vi "Sort References By Type.vi"(10 "Controls to Register":refnum<vi>[](array[refnum])) -> (2 "Controls":T1)   [LabVIEW 2015, in "AutoRegistration.lvlib" / "AutoRegistration.lvclass"]
uses:
  AutoRegistration.lvclass
  Registration References.ctl
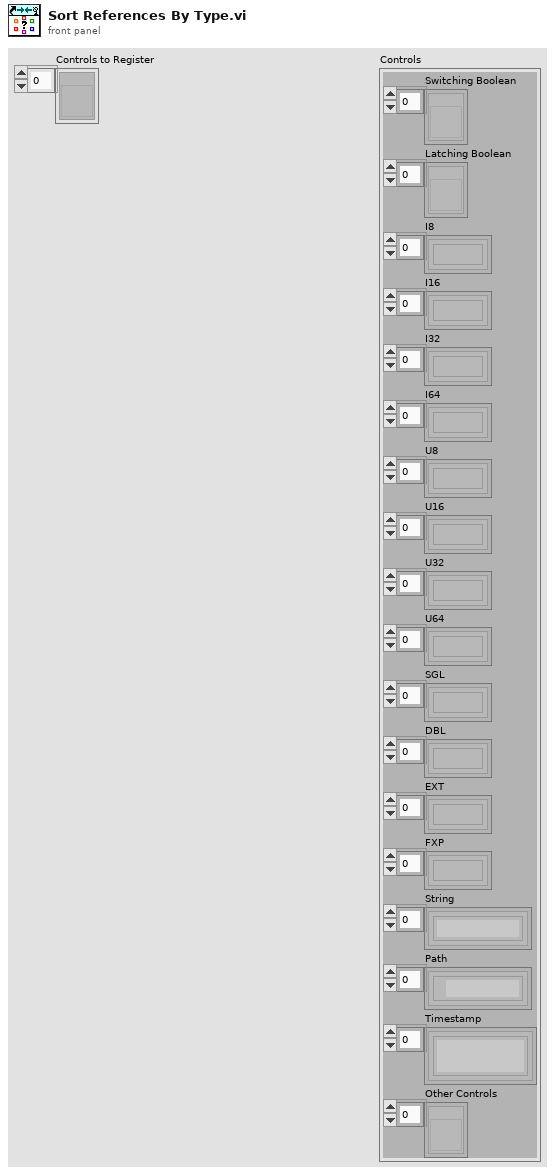
[diagram p1: front panel]
types:
  T1 = typedef "AutoRegistration.lvlib/AutoRegistration.lvclass/Registration References.ctl" = cluster{"Switching Boolean":refnum<vi>[], "Latching Boolean":refnum<vi>[], "I8":refnum<vi>[], "I16":refnum<vi>[], "I32":refnum<vi>[], "I64":refnum<vi>[], "U8":refnum<vi>[], "U16":refnum<vi>[], "U32":refnum<vi>[], "U64":refnum<vi>[], "SGL":refnum<vi>[], "DBL":refnum<vi>[], "EXT":refnum<vi>[], "FXP":refnum<vi>[], "String":refnum<vi>[], "Path":refnum<vi>[], "Timestamp":refnum<vi>[], "Other Controls":refnum<vi>[]}
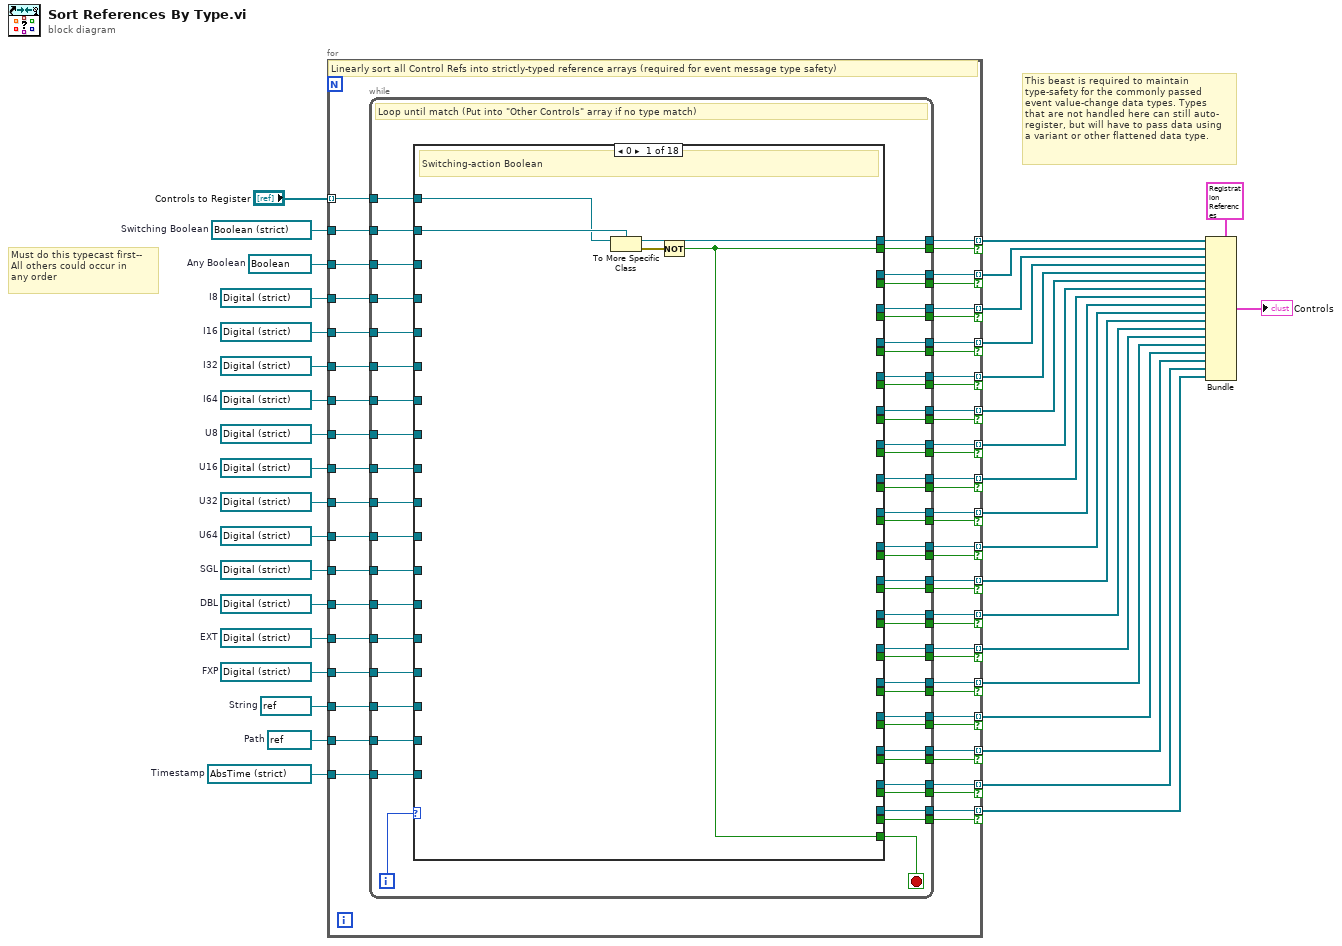
[diagram p0: block diagram]
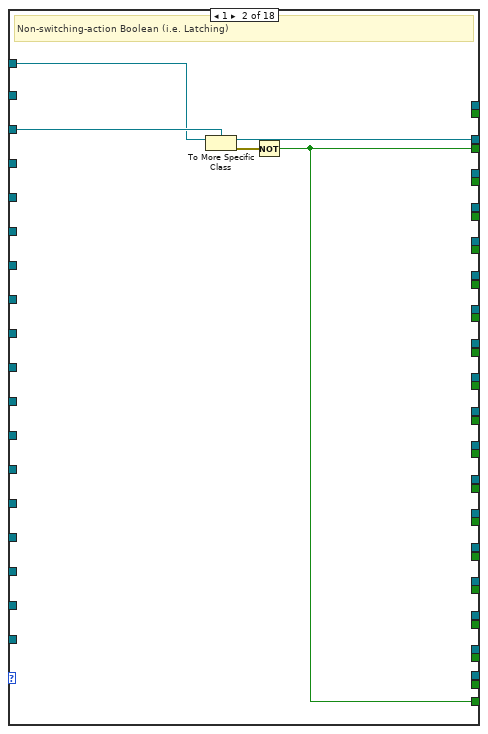
[diagram p2: hidden frame]
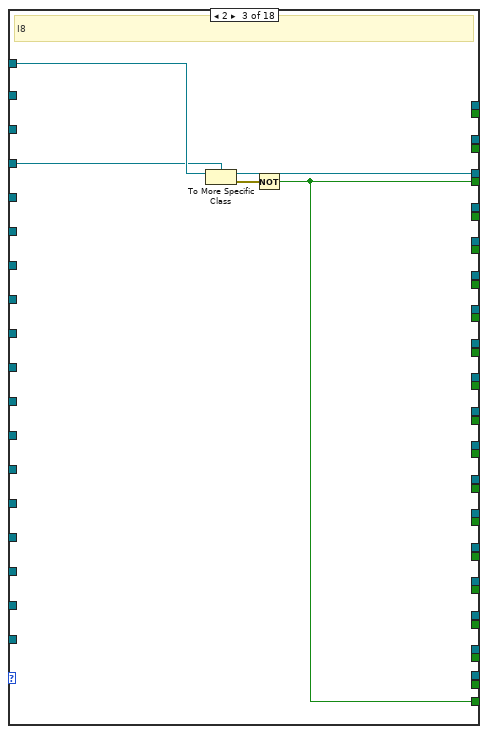
[diagram p3: hidden frame]
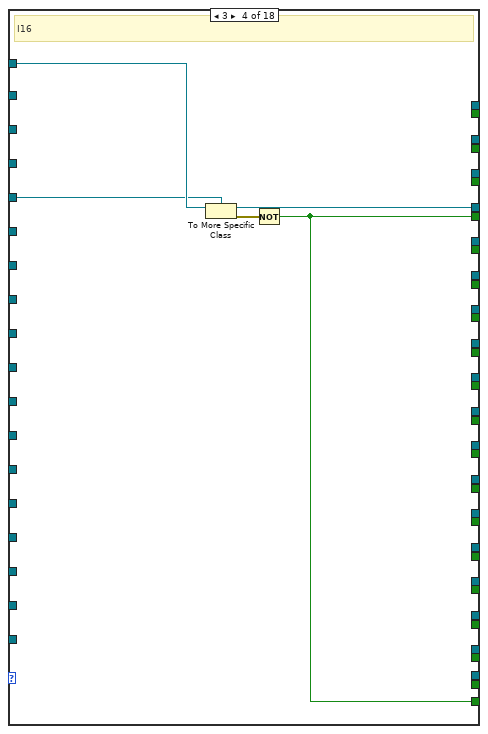
[diagram p4: hidden frame]
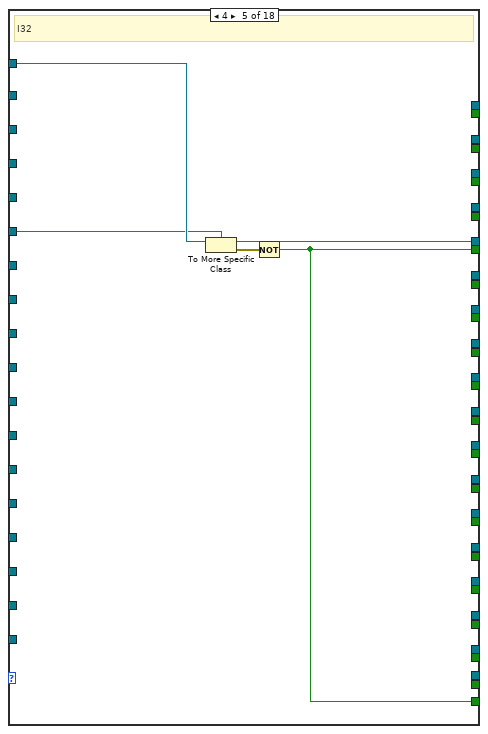
[diagram p5: hidden frame]
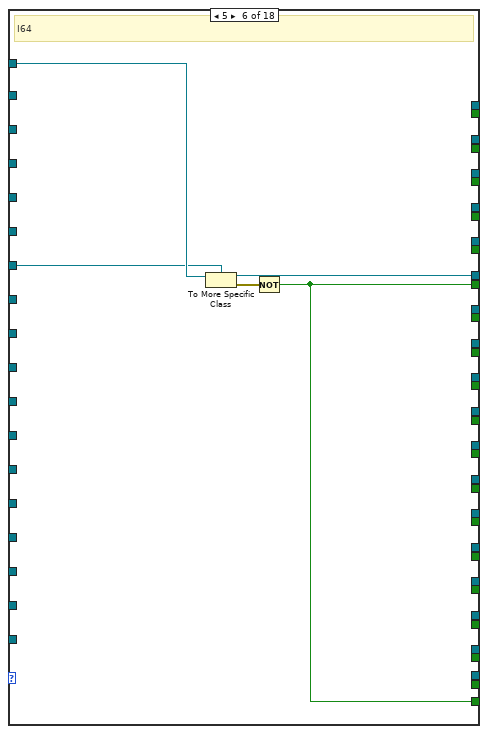
[diagram p6: hidden frame]
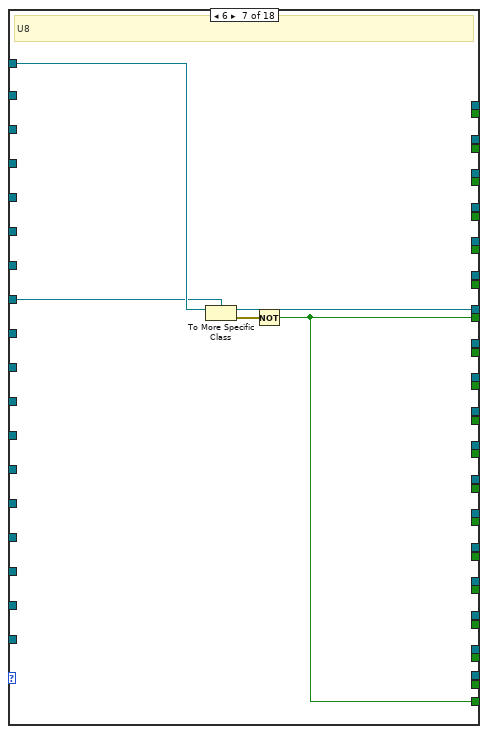
[diagram p7: hidden frame]
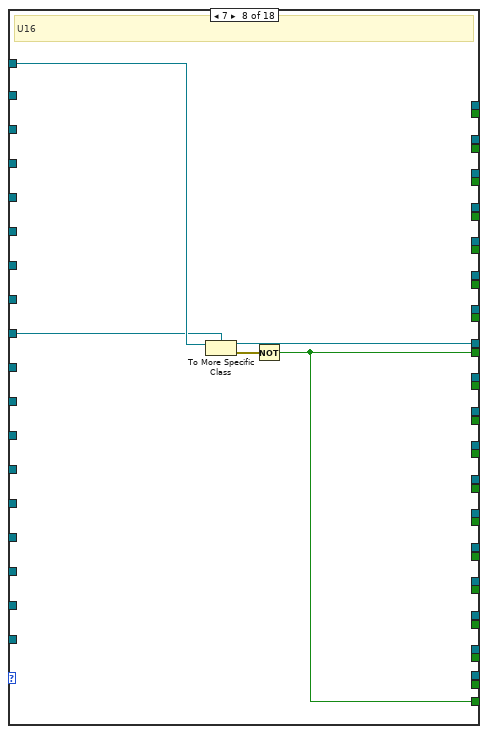
[diagram p8: hidden frame]
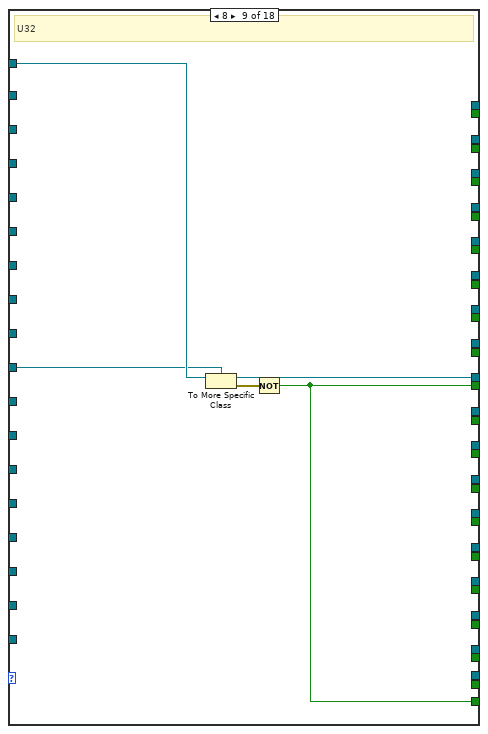
[diagram p9: hidden frame]
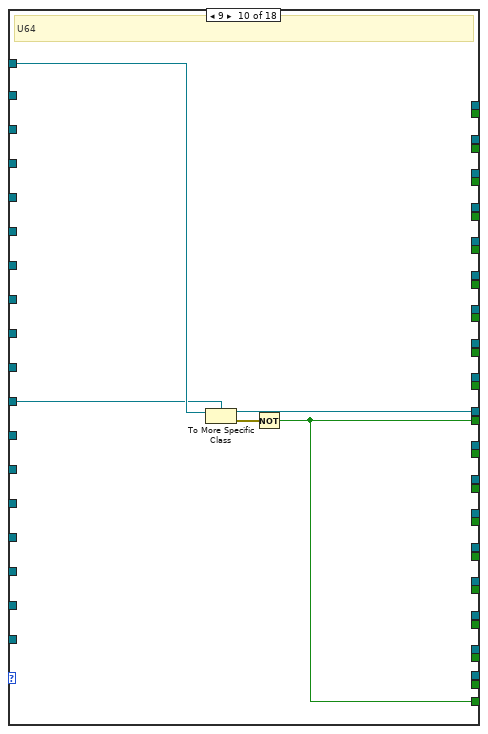
[diagram p10: hidden frame]
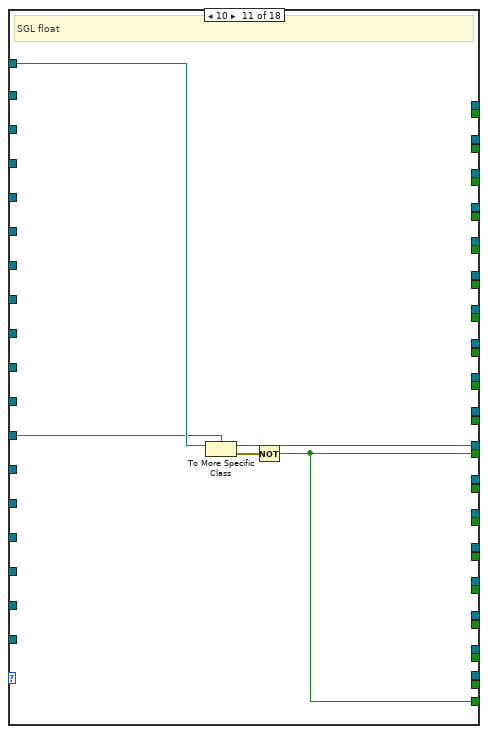
[diagram p11: hidden frame]
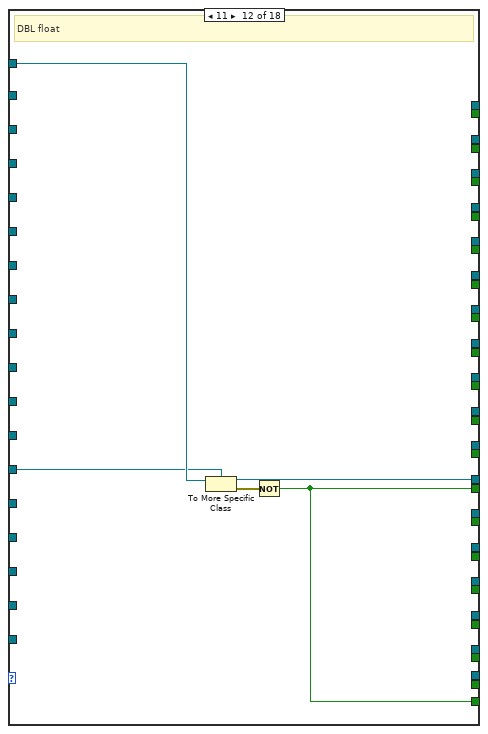
[diagram p12: hidden frame]
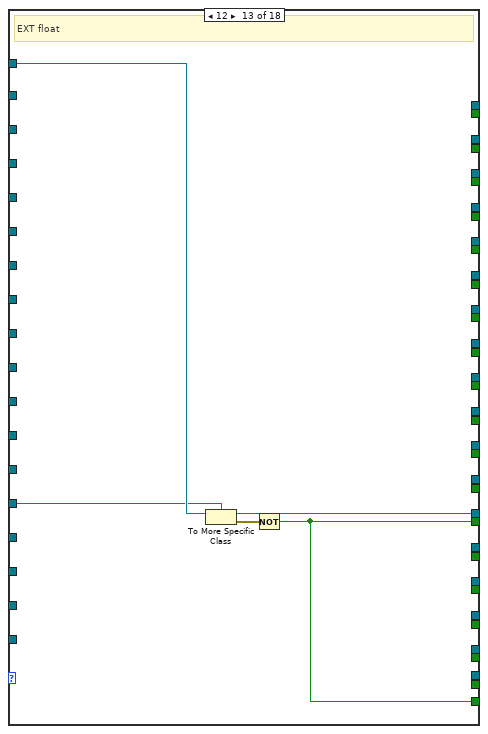
[diagram p13: hidden frame]
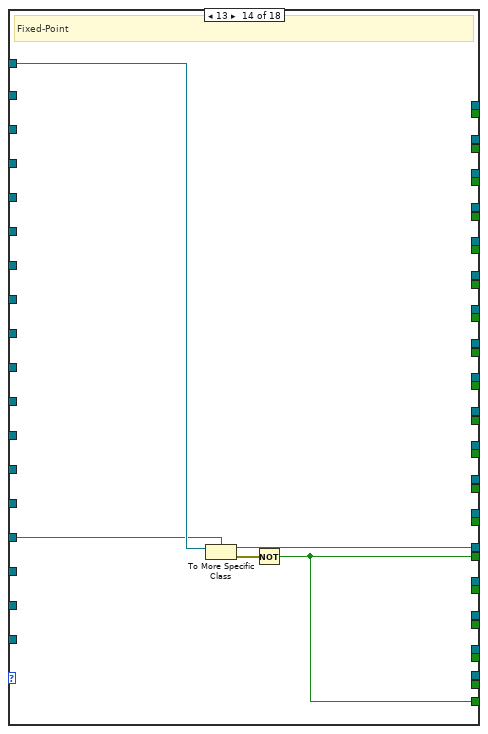
[diagram p14: hidden frame]
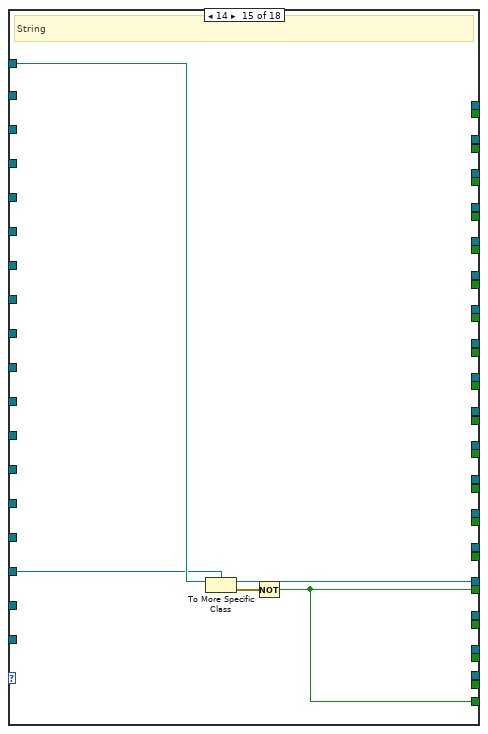
[diagram p15: hidden frame]
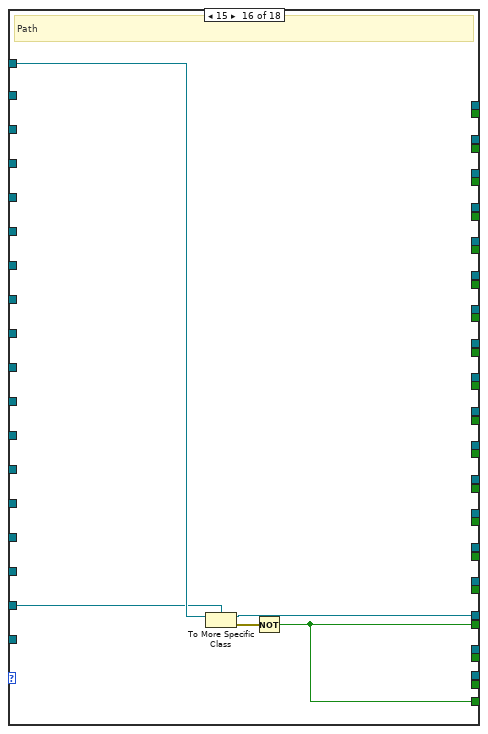
[diagram p16: hidden frame]
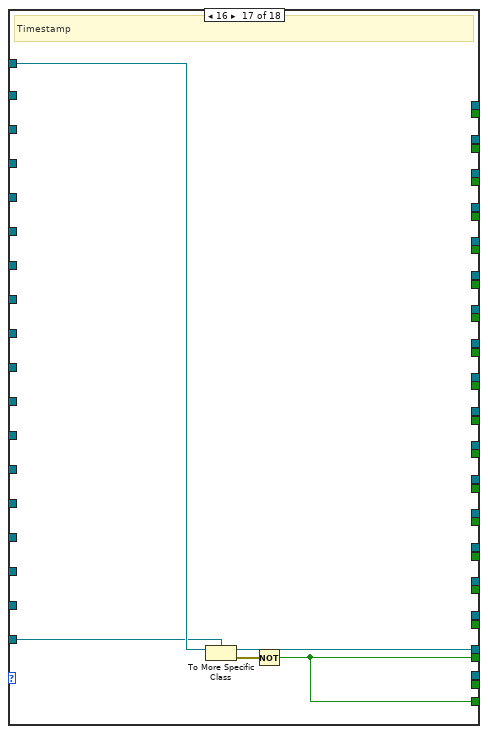
[diagram p17: hidden frame]
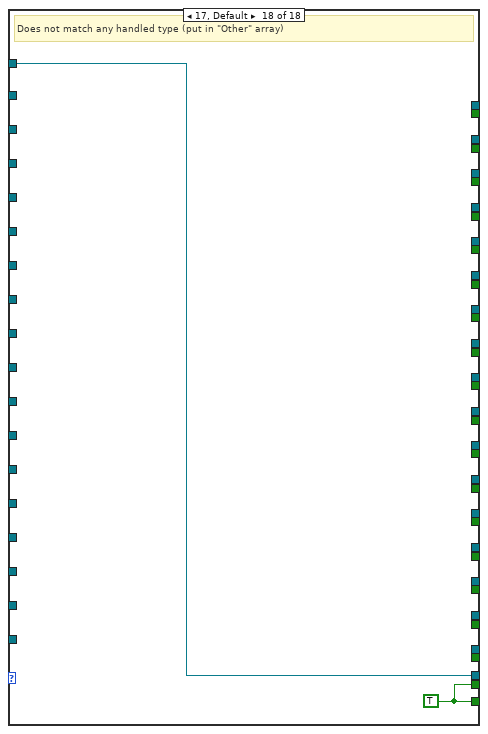
[diagram p18: hidden frame]
diagram:
  w21 = refnum<vi> refnum  # Switching Boolean
  w22 = refnum<vi> refnum  # Any Boolean
  w23 = refnum<vi> refnum  # I8
  w24 = refnum<vi> refnum  # I16
  w25 = refnum<vi> refnum  # I32
  w26 = refnum<vi> refnum  # I64
  w27 = refnum<vi> refnum  # U8
  w28 = refnum<vi> refnum  # U16
  w29 = refnum<vi> refnum  # U32
  w30 = refnum<vi> refnum  # U64
  w31 = refnum<vi> refnum  # SGL
  w32 = refnum<vi> refnum  # DBL
  w33 = refnum<vi> refnum  # EXT
  w34 = refnum<vi> refnum  # FXP
  w35 = refnum<vi> refnum  # String
  w36 = refnum<vi> refnum  # Path
  w37 = refnum<vi> refnum  # Timestamp
  # "Must do this typecast first--\nAll others could occur in\nany order"
  # "This beast is required to maintain\ntype-safety for the commonly passed\nevent value-change data types. Types\nthat are not handled here can still auto-\nregister, but will have to pass data using\na variant or other flattened data type."
  n1 = for {
    tunnel: "Controls to Register" -> [w41] mode=indexing
    tunnel: w37 -> [w92]
    tunnel: w36 -> [w91]
    tunnel: w35 -> [w90]
    tunnel: w34 -> [w89]
    tunnel: w33 -> [w88]
    tunnel: w32 -> [w87]
    tunnel: w31 -> [w86]
    tunnel: w30 -> [w85]
    tunnel: w29 -> [w84]
    tunnel: w28 -> [w83]
    tunnel: w27 -> [w82]
    tunnel: w26 -> [w81]
    tunnel: w25 -> [w80]
    tunnel: w24 -> [w79]
    tunnel: w23 -> [w78]
    tunnel: w22 -> [w77]
    tunnel: w21 -> [w76]
    tunnel: [w75] -> w20 mode=indexing if=w42
    tunnel: [w74] -> w19 mode=indexing if=w58
    tunnel: [w73] -> w18 mode=indexing if=w43
    tunnel: [w72] -> w17 mode=indexing if=w44
    tunnel: [w71] -> w16 mode=indexing if=w45
    tunnel: [w70] -> w15 mode=indexing if=w46
    tunnel: [w69] -> w14 mode=indexing if=w47
    tunnel: [w68] -> w13 mode=indexing if=w48
    tunnel: [w67] -> w12 mode=indexing if=w49
    tunnel: [w66] -> w11 mode=indexing if=w50
    tunnel: [w65] -> w10 mode=indexing if=w51
    tunnel: [w64] -> w9 mode=indexing if=w52
    tunnel: [w63] -> w8 mode=indexing if=w53
    tunnel: [w62] -> w7 mode=indexing if=w54
    tunnel: [w61] -> w6 mode=indexing if=w55
    tunnel: [w60] -> w5 mode=indexing if=w56
    tunnel: [w59] -> w4 mode=indexing if=w57
    tunnel: [w40] -> w3 mode=indexing if=w39
    # "Linearly sort all Control Refs into strictly-typed reference arrays (required for event message type safety)"
    n2 = while {
      tunnel: [w114] -> w58
      tunnel: [w113] -> w57
      tunnel: [w112] -> w56
      tunnel: [w111] -> w55
      tunnel: [w110] -> w54
      tunnel: [w109] -> w53
      tunnel: [w108] -> w52
      tunnel: [w107] -> w51
      tunnel: [w106] -> w50
      tunnel: [w105] -> w49
      tunnel: [w104] -> w48
      tunnel: [w103] -> w47
      tunnel: [w102] -> w46
      tunnel: [w101] -> w45
      tunnel: [w100] -> w44
      tunnel: [w99] -> w43
      tunnel: [w98] -> w42
      tunnel: w41 -> [w97]
      tunnel: w76 -> [w132]
      tunnel: [w131] -> w75
      tunnel: w77 -> [w133]
      tunnel: [w130] -> w74
      tunnel: w78 -> [w134]
      tunnel: [w129] -> w73
      tunnel: w79 -> [w135]
      tunnel: [w128] -> w72
      tunnel: w80 -> [w136]
      tunnel: [w127] -> w71
      tunnel: w81 -> [w137]
      tunnel: [w126] -> w70
      tunnel: w82 -> [w138]
      tunnel: [w125] -> w69
      tunnel: w83 -> [w139]
      tunnel: [w124] -> w68
      tunnel: w84 -> [w140]
      tunnel: [w123] -> w67
      tunnel: w85 -> [w141]
      tunnel: [w122] -> w66
      tunnel: w86 -> [w142]
      tunnel: [w121] -> w65
      tunnel: w87 -> [w143]
      tunnel: [w120] -> w64
      tunnel: w88 -> [w144]
      tunnel: [w119] -> w63
      tunnel: w89 -> [w145]
      tunnel: [w118] -> w62
      tunnel: w90 -> [w146]
      tunnel: [w117] -> w61
      tunnel: w91 -> [w147]
      tunnel: [w116] -> w60
      tunnel: w92 -> [w148]
      tunnel: [w115] -> w59
      tunnel: [w94] -> w40
      tunnel: [w93] -> w39
      i -> [w95]
      stop <- w96 stop-if-true
      # "Loop until match (Put into \"Other Controls\" array if no type match)"
      n3 = case shown="0" w95 {
        tunnel: w148 -> [_ _ _ _ _ _ _ _ _ _ _ _ _ _ _ _ w229 _]
        tunnel: w147 -> [_ _ _ _ _ _ _ _ _ _ _ _ _ _ _ w224 _ _]
        tunnel: w146 -> [_ _ _ _ _ _ _ _ _ _ _ _ _ _ w219 _ _ _]
        tunnel: w145 -> [_ _ _ _ _ _ _ _ _ _ _ _ _ w216 _ _ _ _]
        tunnel: w144 -> [_ _ _ _ _ _ _ _ _ _ _ _ w211 _ _ _ _ _]
        tunnel: w143 -> [_ _ _ _ _ _ _ _ _ _ _ w206 _ _ _ _ _ _]
        tunnel: w142 -> [_ _ _ _ _ _ _ _ _ _ w201 _ _ _ _ _ _ _]
        tunnel: w141 -> [_ _ _ _ _ _ _ _ _ w196 _ _ _ _ _ _ _ _]
        tunnel: w140 -> [_ _ _ _ _ _ _ _ w191 _ _ _ _ _ _ _ _ _]
        tunnel: w139 -> [_ _ _ _ _ _ _ w186 _ _ _ _ _ _ _ _ _ _]
        tunnel: w138 -> [_ _ _ _ _ _ w181 _ _ _ _ _ _ _ _ _ _ _]
        tunnel: w137 -> [_ _ _ _ _ w174 _ _ _ _ _ _ _ _ _ _ _ _]
        tunnel: w136 -> [_ _ _ _ w171 _ _ _ _ _ _ _ _ _ _ _ _ _]
        tunnel: w135 -> [_ _ _ w166 _ _ _ _ _ _ _ _ _ _ _ _ _ _]
        tunnel: w134 -> [_ _ w160 _ _ _ _ _ _ _ _ _ _ _ _ _ _ _]
        tunnel: w133 -> [_ w158 _ _ _ _ _ _ _ _ _ _ _ _ _ _ _ _]
        tunnel: w132 -> [w153 _ _ _ _ _ _ _ _ _ _ _ _ _ _ _ _ _]
        tunnel: [w152 _ _ _ _ _ _ _ _ _ _ _ _ _ _ _ _ _] -> w131
        tunnel: [_ w154 _ _ _ _ _ _ _ _ _ _ _ _ _ _ _ _] -> w130
        tunnel: [_ _ w159 _ _ _ _ _ _ _ _ _ _ _ _ _ _ _] -> w129
        tunnel: [_ _ _ w165 _ _ _ _ _ _ _ _ _ _ _ _ _ _] -> w128
        tunnel: [_ _ _ _ w169 _ _ _ _ _ _ _ _ _ _ _ _ _] -> w127
        tunnel: [_ _ _ _ _ w175 _ _ _ _ _ _ _ _ _ _ _ _] -> w126
        tunnel: [_ _ _ _ _ _ w179 _ _ _ _ _ _ _ _ _ _ _] -> w125
        tunnel: [_ _ _ _ _ _ _ w184 _ _ _ _ _ _ _ _ _ _] -> w124
        tunnel: [_ _ _ _ _ _ _ _ w189 _ _ _ _ _ _ _ _ _] -> w123
        tunnel: [_ _ _ _ _ _ _ _ _ w194 _ _ _ _ _ _ _ _] -> w122
        tunnel: [_ _ _ _ _ _ _ _ _ _ w199 _ _ _ _ _ _ _] -> w121
        tunnel: [_ _ _ _ _ _ _ _ _ _ _ w204 _ _ _ _ _ _] -> w120
        tunnel: [_ _ _ _ _ _ _ _ _ _ _ _ w209 _ _ _ _ _] -> w119
        tunnel: [_ _ _ _ _ _ _ _ _ _ _ _ _ w214 _ _ _ _] -> w118
        tunnel: [_ _ _ _ _ _ _ _ _ _ _ _ _ _ w220 _ _ _] -> w117
        tunnel: [_ _ _ _ _ _ _ _ _ _ _ _ _ _ _ w225 _ _] -> w116
        tunnel: [_ _ _ _ _ _ _ _ _ _ _ _ _ _ _ _ w230 _] -> w115
        tunnel: [_ w155 _ _ _ _ _ _ _ _ _ _ _ _ _ _ _ _] -> w114
        tunnel: [_ _ _ _ _ _ _ _ _ _ _ _ _ _ _ _ w231 _] -> w113
        tunnel: [_ _ _ _ _ _ _ _ _ _ _ _ _ _ _ w226 _ _] -> w112
        tunnel: [_ _ _ _ _ _ _ _ _ _ _ _ _ _ w221 _ _ _] -> w111
        tunnel: [_ _ _ _ _ _ _ _ _ _ _ _ _ w215 _ _ _ _] -> w110
        tunnel: [_ _ _ _ _ _ _ _ _ _ _ _ w210 _ _ _ _ _] -> w109
        tunnel: [_ _ _ _ _ _ _ _ _ _ _ w205 _ _ _ _ _ _] -> w108
        tunnel: [_ _ _ _ _ _ _ _ _ _ w200 _ _ _ _ _ _ _] -> w107
        tunnel: [_ _ _ _ _ _ _ _ _ w195 _ _ _ _ _ _ _ _] -> w106
        tunnel: [_ _ _ _ _ _ _ _ w190 _ _ _ _ _ _ _ _ _] -> w105
        tunnel: [_ _ _ _ _ _ _ w185 _ _ _ _ _ _ _ _ _ _] -> w104
        tunnel: [_ _ _ _ _ _ w180 _ _ _ _ _ _ _ _ _ _ _] -> w103
        tunnel: [_ _ _ _ _ w176 _ _ _ _ _ _ _ _ _ _ _ _] -> w102
        tunnel: [_ _ _ _ w170 _ _ _ _ _ _ _ _ _ _ _ _ _] -> w101
        tunnel: [_ _ _ w164 _ _ _ _ _ _ _ _ _ _ _ _ _ _] -> w100
        tunnel: [_ _ w161 _ _ _ _ _ _ _ _ _ _ _ _ _ _ _] -> w99
        tunnel: [w149 _ _ _ _ _ _ _ _ _ _ _ _ _ _ _ _ _] -> w98
        tunnel: w97 -> [w150 w156 w162 w167 w172 w177 w182 w187 w192 w197 w202 w207 w212 w217 w222 w227 w232 w235]
        tunnel: [w149 w155 w161 w164 w170 w176 w180 w185 w190 w195 w200 w205 w210 w215 w221 w226 w231 w234] -> w96
        tunnel: [_ _ _ _ _ _ _ _ _ _ _ _ _ _ _ _ _ w235] -> w94
        tunnel: [_ _ _ _ _ _ _ _ _ _ _ _ _ _ _ _ _ w234] -> w93
        frame 0 {
          # "Switching-action Boolean"
          n4 = To More Specific Class(target class=w153, reference=w150) -> (specific class reference=w152:refnum<vi>, error out=w151:errorcluster)  [unwired: 1 in]
          n5 = Not(x=w151) -> (.not. x?=w149:bool)
        }
        frame 1 {
          # "Non-switching-action Boolean (i.e. Latching)"
          n6 = To More Specific Class(target class=w158, reference=w156) -> (specific class reference=w154:refnum<vi>, error out=w157:errorcluster)  [unwired: 1 in]
          n7 = Not(x=w157) -> (.not. x?=w155:bool)
        }
        frame 2 {
          # "I8"
          n8 = To More Specific Class(target class=w160, reference=w162) -> (specific class reference=w159:refnum<vi>, error out=w163:errorcluster)  [unwired: 1 in]
          n9 = Not(x=w163) -> (.not. x?=w161:bool)
        }
        frame 3 {
          # "I16"
          n10 = To More Specific Class(target class=w166, reference=w167) -> (specific class reference=w165:refnum<vi>, error out=w168:errorcluster)  [unwired: 1 in]
          n11 = Not(x=w168) -> (.not. x?=w164:bool)
        }
        frame 4 {
          # "I32"
          n12 = To More Specific Class(target class=w171, reference=w172) -> (specific class reference=w169:refnum<vi>, error out=w173:errorcluster)  [unwired: 1 in]
          n13 = Not(x=w173) -> (.not. x?=w170:bool)
        }
        frame 5 {
          # "I64"
          n14 = To More Specific Class(target class=w174, reference=w177) -> (specific class reference=w175:refnum<vi>, error out=w178:errorcluster)  [unwired: 1 in]
          n15 = Not(x=w178) -> (.not. x?=w176:bool)
        }
        frame 6 {
          # "U8"
          n16 = To More Specific Class(target class=w181, reference=w182) -> (specific class reference=w179:refnum<vi>, error out=w183:errorcluster)  [unwired: 1 in]
          n17 = Not(x=w183) -> (.not. x?=w180:bool)
        }
        frame 7 {
          # "U16"
          n18 = To More Specific Class(target class=w186, reference=w187) -> (specific class reference=w184:refnum<vi>, error out=w188:errorcluster)  [unwired: 1 in]
          n19 = Not(x=w188) -> (.not. x?=w185:bool)
        }
        frame 8 {
          # "U32"
          n20 = To More Specific Class(target class=w191, reference=w192) -> (specific class reference=w189:refnum<vi>, error out=w193:errorcluster)  [unwired: 1 in]
          n21 = Not(x=w193) -> (.not. x?=w190:bool)
        }
        frame 9 {
          # "U64"
          n22 = To More Specific Class(target class=w196, reference=w197) -> (specific class reference=w194:refnum<vi>, error out=w198:errorcluster)  [unwired: 1 in]
          n23 = Not(x=w198) -> (.not. x?=w195:bool)
        }
        frame 10 {
          # "SGL float"
          n24 = To More Specific Class(target class=w201, reference=w202) -> (specific class reference=w199:refnum<vi>, error out=w203:errorcluster)  [unwired: 1 in]
          n25 = Not(x=w203) -> (.not. x?=w200:bool)
        }
        frame 11 {
          # "DBL float"
          n26 = To More Specific Class(target class=w206, reference=w207) -> (specific class reference=w204:refnum<vi>, error out=w208:errorcluster)  [unwired: 1 in]
          n27 = Not(x=w208) -> (.not. x?=w205:bool)
        }
        frame 12 {
          # "EXT float"
          n28 = To More Specific Class(target class=w211, reference=w212) -> (specific class reference=w209:refnum<vi>, error out=w213:errorcluster)  [unwired: 1 in]
          n29 = Not(x=w213) -> (.not. x?=w210:bool)
        }
        frame 13 {
          # "Fixed-Point"
          n30 = To More Specific Class(target class=w216, reference=w217) -> (specific class reference=w214:refnum<vi>, error out=w218:errorcluster)  [unwired: 1 in]
          n31 = Not(x=w218) -> (.not. x?=w215:bool)
        }
        frame 14 {
          # "String"
          n32 = To More Specific Class(target class=w219, reference=w222) -> (specific class reference=w220:refnum<vi>, error out=w223:errorcluster)  [unwired: 1 in]
          n33 = Not(x=w223) -> (.not. x?=w221:bool)
        }
        frame 15 {
          # "Path"
          n34 = To More Specific Class(target class=w224, reference=w227) -> (specific class reference=w225:refnum<vi>, error out=w228:errorcluster)  [unwired: 1 in]
          n35 = Not(x=w228) -> (.not. x?=w226:bool)
        }
        frame 16 {
          # "Timestamp"
          n36 = To More Specific Class(target class=w229, reference=w232) -> (specific class reference=w230:refnum<vi>, error out=w233:errorcluster)  [unwired: 1 in]
          n37 = Not(x=w233) -> (.not. x?=w231:bool)
        }
        frame 17, Default {
          w234 = TRUE
          # "Does not match any handled type (put in \"Other\" array)"
        }
      }
    }
  }
  n38 = Bundle(cluster=T1 {"Switching Boolean"=[], "Latching Boolean"=[], "I8"=[], "I16"=[], "I32"=[], "I64"=[], "U8"=[], "U16"=[], "U32"=[], "U64"=[], "SGL"=[], "DBL"=[], "EXT"=[], "FXP"=[], "String"=[], "Path"=[], "Timestamp"=[], "Other Controls"=[]} ("Controls"), "Switching Boolean"=w20, "Latching Boolean"=w19, "I8"=w18, "I16"=w17, "I32"=w16, "I64"=w15, "U8"=w14, "U16"=w13, "U32"=w12, "U64"=w11, "SGL"=w10, "DBL"=w9, "EXT"=w8, "FXP"=w7, "String"=w6, "Path"=w5, "Timestamp"=w4, "Other Controls"=w3) -> (→"Controls":T1)
